vi "启动vi(显示登录) .vi"   [LabVIEW 2015]
panel:
  # "点击运行启动"
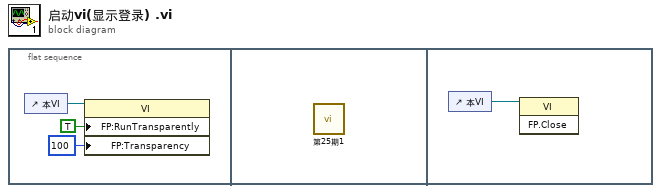
[diagram p0: block diagram]
diagram:
  n1 = flat-sequence {
    frame #0 {
      n2 = control-ref of="本VI"() -> (w1:refnum<vi>)
      n3 = property class="VI"(reference=w1, "FP:RunTransparently"=TRUE ("前面板窗口:以透明方式运行VI"), "FP:Transparency"=u8 100 ("前面板窗口:透明度")) -> ()  [unwired: 1 in, 2 out]
    }
    frame #1 {
      n4 = call "第25期1.vi"() -> ()  [unwired: 11 in, 1 out]
    }
    frame #2 {
      n5 = control-ref of="本VI"() -> (w4:refnum<vi>)
      n6 = invoke class="VI" method="FP.Close"(reference=w4) -> ()  [unwired: 2 in, 3 out]
    }
  }
